vi "IDtoSubnodeclass.vi"(8 "error in (no error)":errorcluster, 11 "Navigate Tree:Get Parent":string) -> (0 "error out":errorcluster, 1 "invalid Id":bool, 2 "subnodes class":string[](array[string]), 3 "node ref":T1)   [LabVIEW 2025, in "CEF.lvlib" / "CEF_Node.lvclass"]
doc: "Copyright 2017 National Instruments Corporation\n\nLicensed under the Apache License, Version 2.0 (the \"License\"); you may not use this file except in compliance with the License. You may obtain a copy of the License at http://www.apache.org/licenses/LICENSE-2.0\nUnless required by applicable law or agreed to in writing, software distributed under the License is distributed on an \"AS IS\" BASIS, WITHOUT WARRANTIES OR CONDITIONS OF ANY KIND, either express or implied. See the License for the specific language governing permissions and limitations under the License."
uses:
  CEF_Node.lvclass
  NodeRef.ctl
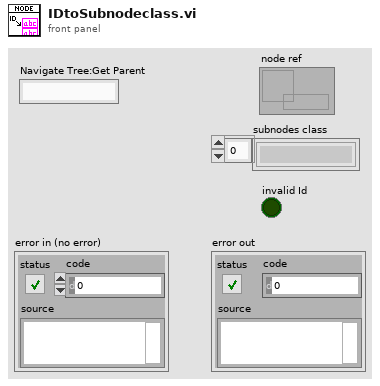
[diagram p1: front panel]
types:
  T1 = typedef "CEF.lvlib/CEF_Node.lvclass/NodeRef.ctl" = refnum<data-value>
  T2 = typedef "CEF.lvlib/CEF_Node.lvclass/SubNodeCluster.ctl" = cluster{"subnodes menu name":string[], "subnodes class":string[], "subnodes category":string[]}
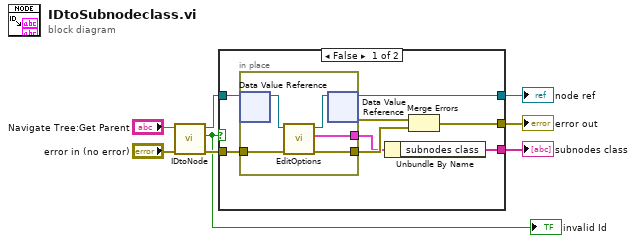
[diagram p0: block diagram]
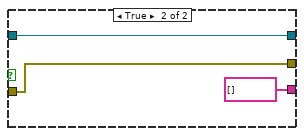
[diagram p2: hidden frame]
diagram:
  n1 = call "IDtoNode.vi"("error in"="error in (no error)", "ID"="Navigate Tree:Get Parent") -> ("error out"=w4:errorcluster, "invalid Id"=w3:bool, "node ref"=w2:T1)  [unwired: 7 in]
  "invalid Id" <- w3
  n2 = case shown="False" w3 {
    tunnel: w2 -> [w16 w22]
    tunnel: [w10 string[] [] ("subnodes class")] -> w5
    tunnel: w4 -> [w15 w24]
    tunnel: [w12 w24] -> w8
    tunnel: [w9 w22] -> w1
    frame False {
      n3 = in-place {
        in-place-border: [w19] -> w11
        in-place-border: w15 -> [w18]
        in-place-border: [w17] -> w14
        n4 = in-place-dvr #1(w16) -> (w21:refnum<class "CEF_Node.lvclass">)  [unwired: 1 out]
        n5 = call-dynamic "EditOptions.vi"("error in"=w18, "CEF_Node in"=w21) -> ("error out"=w17:errorcluster, "subnodes class"=w19:T2, "CEF_Node out"=w20:refnum<class "CEF_Node.lvclass">)  [unwired: 6 in, 1 out]
        n6 = in-place-dvr #1(w20) -> (w9:T1, w13:errorcluster)
      }
      n7 = Unbundle By Name(w11) -> ("subnodes class"=w10:string[])
      n8 = Merge Errors(w13, w14) -> (w12:errorcluster)
    }
    frame True {
    }
  }
  "error out" <- w8
  "subnodes class" <- w5
  "node ref" <- w1
